vi "Remove Section.vi"(7 "section":string, 8 "error in (no error)":errorcluster, 11 "refnum":T1) -> (0 "error out":errorcluster, 2 "section exists?":bool, 3 "refnum out":T1)   [LabVIEW 2017, in "NI_LVConfig.lvlib"]
doc: "Removes a section from the configuration data identified by <B>refnum</B>."
uses:
  <vilib>/Utility/config.llb/NI_LVConfig.lvlib
  <vilib>/Utility/config.llb/Config Data RefNum.ctl
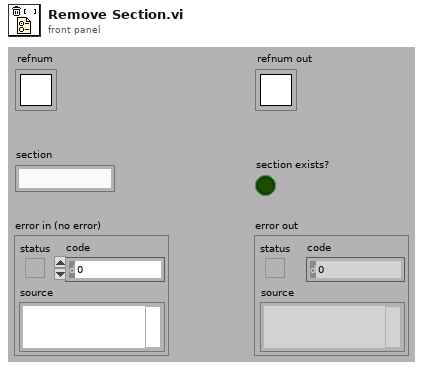
[diagram p1: front panel]
types:
  T1 = typedef "NI_LVConfig.lvlib/Config Data RefNum.ctl" = refnum<k1>
  T2 = typedef "NI_LVConfig.lvlib/Config Queue.ctl" = refnum<queue>
  T3 = typedef "NI_LVConfig.lvlib/Config Data.ctl" = cluster{"sections":T4[], "path":path, "dirty":bool}
  T4 = typedef "NI_LVConfig.lvlib/Section.ctl" = cluster{"name":string, "comment":string, "kvc":string[][]}
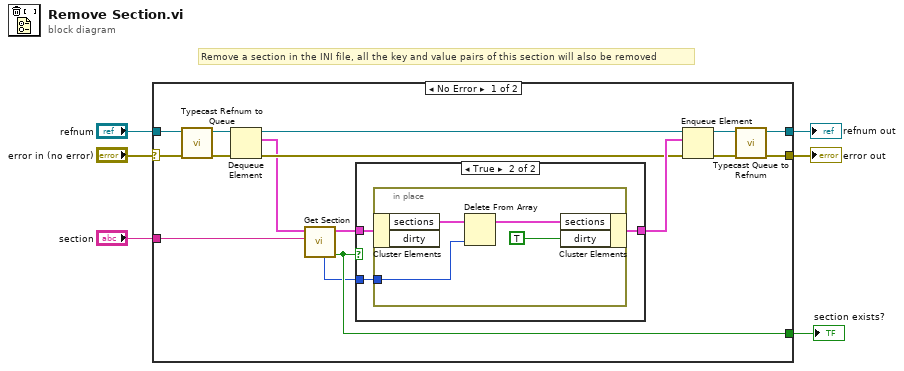
[diagram p0: block diagram]
diagram:
  # "Remove a section in the INI file, all the key and value pairs of this section will also be removed"
  n1 = case shown="No Error" "error in (no error)" {
    selector: "error in (no error)" -> [w12 w30]
    tunnel: [w17 w30] -> w1
    tunnel: [w14 w29] -> w3
    tunnel: "refnum" -> [w16 w29]
    tunnel: "section" -> [w10 _]
    tunnel: [w9 _] -> w2
    frame No Error {
      n2 = call <vilib>:"Typecast Refnum to Queue.vi"("refnum in"=w16) -> ("queue out"=w13:T2)  [unwired: 10 out]
      n3 = Dequeue Element(queue=w13, error in (no error)=w12) -> (queue out=w19:T2, element=w11:T3, error out=w18:errorcluster)  [unwired: 2 out]
      n4 = call <vilib>:"Get Section.vi"("section"=w10, "element"=w11) -> ("section exists?"=w9:bool, "element out"=w8:T3, "section index"=w7:i32)  [unwired: 2 in, 5 out]
      n5 = case shown="True" w9 {
        tunnel: [w21 w24] -> w20
        tunnel: w7 -> [_ w23]
        tunnel: w8 -> [w21 w22]
        frame False {
        }
        frame True {
          n6 = in-place {
            in-place-border: w23 -> [w28]
            n7 = in-place-cluster #1(w22) -> ("sections"=w27:T4[])  [unwired: 1 out]
            n8 = Delete From Array(array=w27, index=w28) -> (array with subset deleted=w26:T4[])  [unwired: 1 in, 1 out]
            n9 = in-place-cluster #1("sections"=w26, "dirty"=TRUE) -> (w24:T3)
          }
        }
      }
      n10 = Enqueue Element(queue=w19, element=w20, error in (no error)=w18) -> (queue out=w15:T2, error out=w17:errorcluster)  [unwired: 2 out]
      n11 = call <vilib>:"Typecast Queue to Refnum.vi"("queue in"=w15) -> ("refnum out"=w14:T1)  [unwired: 10 out]
    }
    frame Error {
    }
  }
  "error out" <- w1
  "section exists?" <- w2
  "refnum out" <- w3
